vi "driveable path calculation test (host).vi"() -> ()   [LabVIEW 2009]
uses:
  <vilib>/rvi/interface/nirviOpenFPGA/nirviOpenFPGA.xnode
  FPGA Bitfiles/Athena Brain.lvproj_FPGA Target 2_driveable path cal~F0.lvbitx
  driveable path calculation.vi
  <vilib>/userDefined/High Color/nirio_resource_hc.ctl
  <vilib>/rvi/interface/nirviCloseFPGA/nirviCloseFPGA.xnode
  <vilib>/rvi/interface/nirviReadWriteControl/nirviReadWriteControl.xnode
  <vilib>/RVI Host/nirviSupport.llb/nirviErrorClusterFromErrorCode.vi
  <vilib>/rvi/errors/niLvFpgaWhatHappensToTopLevelVI.ctl
  <vilib>/rvi/interface/common/niFpgaNodeNameForErrorReporting.ctl
  <vilib>/rvi/errors/niLvFpgaAdjustHostInterfaceError.vi
  <vilib>/FPGAPlugInAG/sbRIO-9642/nirviIntfClose_sbRIO-9642.vi
panel:
  in  "stop":bool
  out "driveable path lengths":u16[](array[numeric])
  out "XY Graph":T1(graph)
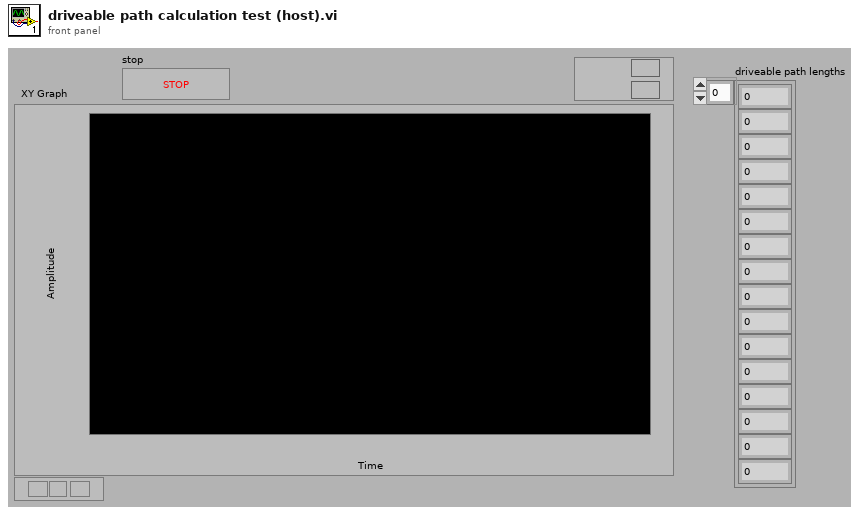
[diagram p1: front panel]
types:
  T1 = cluster{"New X Position":i16, "New Y Position":i16}[]
  T2 = typedef "niFpgaNodeNameForErrorReporting.ctl" = enum16{"Open FPGA VI Reference", "Read/Write Control", "Invoke Method: Abort", "Invoke Method: Acknowledge IRQ", "Invoke Method: Download", "Invoke Method: FIFO.Configure", "Invoke Method: FIFO.Read", "Invoke Method: FIFO.Start", "Invoke Method: FIFO.Stop", "Invoke Method: FIFO.Write", "Invoke Method: Reset", "Invoke Method: Run", "Invoke Method: Wait on IRQ", "Close FPGA VI Reference"}
  T3 = typedef "niLvFpgaWhatHappensToTopLevelVI.ctl" = enum16{"top level VI scripted behind XNode", "top level VI inlined behind XNode"}
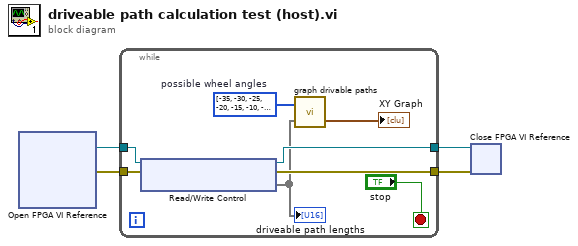
[diagram p0: block diagram]
diagram:
  n1 = xnode "Open FPGA VI Reference"() -> ("FPGA VI Reference Out"=w2:refnum<k20>, "error out"=w1:errorcluster)  [unwired: 2 in]
  n2 = while {
    tunnel: [w12] -> w4
    tunnel: [w11] -> w3
    tunnel: w2 -> [w8]
    tunnel: w1 -> [w7]
    stop <- "stop" stop-if-true
    w9 = i8[] [-35, -30, -25, -20, -15, -10, -5, -1, 1, 5, 10, 15, 20, 25, 30, 35]  # possible wheel angles
    n3 = xnode "Read/Write Control"("FPGA VI Reference In"=w8, "error in"=w7) -> ("FPGA VI Reference Out"=w12:refnum<k20>, "error out"=w11:errorcluster, "driveable path lengths"=w10:void[])
    "driveable path lengths" <- w10
    n4 = call "graph drivable paths.vi"("updated max path lengths"=w10, "possible wheel angles"=w9) -> ("XY Graph"=→"XY Graph":T1)  [unwired: 1 in]
  }
  n5 = xnode "Close FPGA VI Reference"("FPGA VI Reference In"=w4, "error in"=w3) -> ()  [unwired: 1 out]
